vi "LCB Read Event.vi"(8 "error in (no error)":errorcluster caption="Fehler (Eingang, kein Fehler)") -> (0 "error out":errorcluster caption="Fehler (Ausgang)", 1 "Data 2":i32, 2 "Data 1":i32, 3 "Event Identifier":i32, 5 "Data 3":i32)   [LabVIEW 2021, in "labbCAN_Bus_API.lvlib"]
doc: "LCB_Func long __stdcall LCB_ReadEvent(long *pEventId,\n long *pData1,\n long *pData2,\n long *pData3);"
uses:
  labbCAN_Bus_API.lvlib
  labbCAN_Bus_API.dll
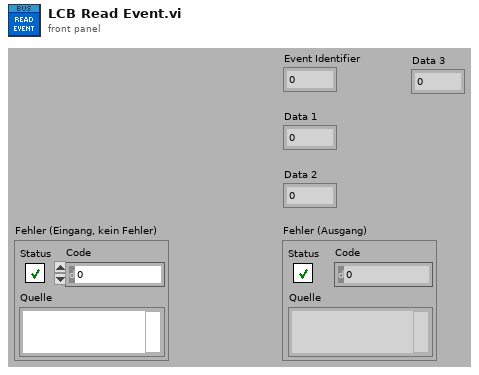
[diagram p1: front panel]
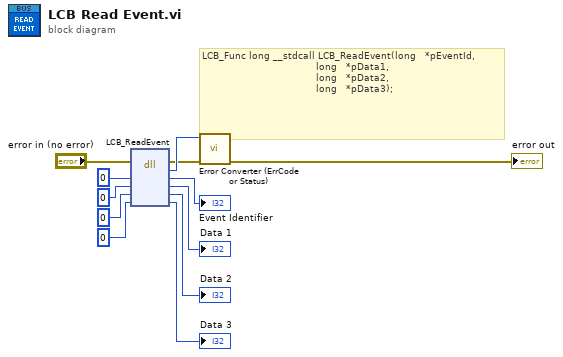
[diagram p0: block diagram]
diagram:
  # "LCB_Func long __stdcall LCB_ReadEvent(long   *pEventId,\n                                      long   *pData1,\n                                      long   *pData2,\n                                      long   *pData3);"
  n1 = dll-call lib="C:/Users/olaja/AppData/Local/CETONI_SDK/labbCAN_Bus_API.*" fn="LCB_ReadEvent"(error in="error in (no error)", "pEventId"=0, "pData1"=0, "pData2"=0, "pData3"=0) -> (error out=w2:errorcluster, w3:i32, "pEventId"=→"Event Identifier":i32, "pData1"=→"Data 1":i32, "pData2"=→"Data 2":i32, "pData3"=→"Data 3":i32)  [unwired: 2 in, 1 out]
  n2 = call "Error Converter (ErrCode or Status).vi"("error in (no error)"=w2, "error code"=w3) -> ("error out"=→"error out":errorcluster)  [unwired: 9 in]
